vi "runCommand.vi"(1 "command":string) -> ()   [LabVIEW 2020]
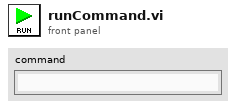
[diagram p1: front panel]
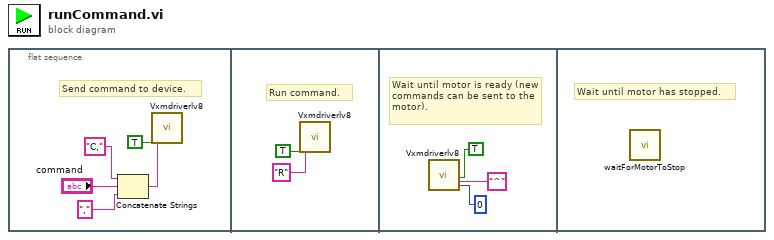
[diagram p0: block diagram]
diagram:
  n1 = flat-sequence {
    frame #0 {
      # "Send command to device."
      n2 = Concatenate Strings("C," ("string"), "command", "," ("string")) -> (w2:string)
      n3 = call "Vxmdriverlv8.Vi"("Send\nchars\nto port"=TRUE ("Send\nchars\nto port"), "Chars to send"=w2) -> ()  [unwired: 20 in, 6 out]
    }
    frame #1 {
      # "Run command."
      n4 = call "Vxmdriverlv8.Vi"("Send\nchars\nto port"=TRUE ("Send\nchars\nto port"), "Chars to send"="R") -> ()  [unwired: 20 in, 6 out]
    }
    frame #2 {
      # "Wait until motor is ready (new commands can be sent to the motor)."
      n5 = call "Vxmdriverlv8.Vi"("Wait\nfor \nchar"=TRUE ("Wait\nfor \nchar"), "Char(s) to wait for"="^", "Char\nTimeout\nTime (ms)"=0 ("Char\nTimeout\nTime (ms)")) -> ()  [unwired: 19 in, 6 out]
    }
    frame #3 {
      # "Wait until motor has stopped."
      n6 = call "waitForMotorToStop.vi"() -> ()  [unwired: 1 in]
    }
  }
